vi "Read U16.vi"(6 "timeout ms (1000)":i32=1000, 7 "Function Code":u8, 8 "error in (no error)":errorcluster, 9 "Number of Registers":u16, 10 "Start Address":u16, 11 "TCP Network Connection in":refnum<k5>) -> (0 "error out":errorcluster, 2 "Results":u16[](array[numeric]), 3 "TCP Network Connection out":refnum<k5>)   [LabVIEW 2023, in "Modbus TCP Micro.lvlib"]
uses:
  Modbus TCP Micro.lvlib
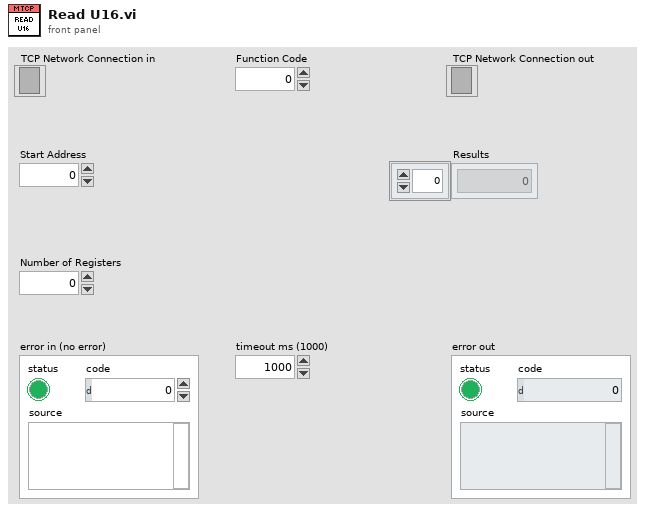
[diagram p1: front panel]
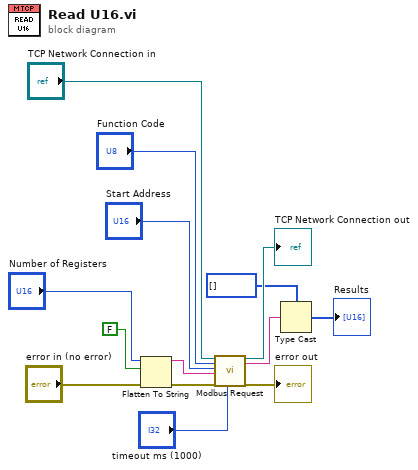
[diagram p0: block diagram]
diagram:
  n1 = Flatten To String(anything="Number of Registers", prepend array or string size? (T)=FALSE, error in (no error)="error in (no error)") -> (data string=w4:string, error out=w7:errorcluster)  [unwired: 1 in, 1 out]
  n2 = call "Modbus Request.vi"("TCP Network Connection in"="TCP Network Connection in", "Function Codes"="Function Code", "Start Address"="Start Address", "Payload"=w4, "error in (no error)"=w7, "timeout ms (1000)"="timeout ms (1000)") -> ("TCP Network Connection out"=→"TCP Network Connection out":refnum<k5>, "Payload"=w10:string, "error out"=→"error out":errorcluster)  [unwired: 8 in, 3 out]
  n3 = Type Cast(type=u16[] [], x=w10) -> (*(type *) &x=→"Results":u16[])
